vi "Прием ОС (SubVI).vi"(10 "Адрес ОУ":u8, 11 "RX Data":bool[](array[boolean])) -> (2 "Признаки":bool[](array[boolean]), 3 "Ошибка ОС":bool)   [LabVIEW 2015]
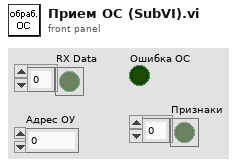
[diagram p1: front panel]
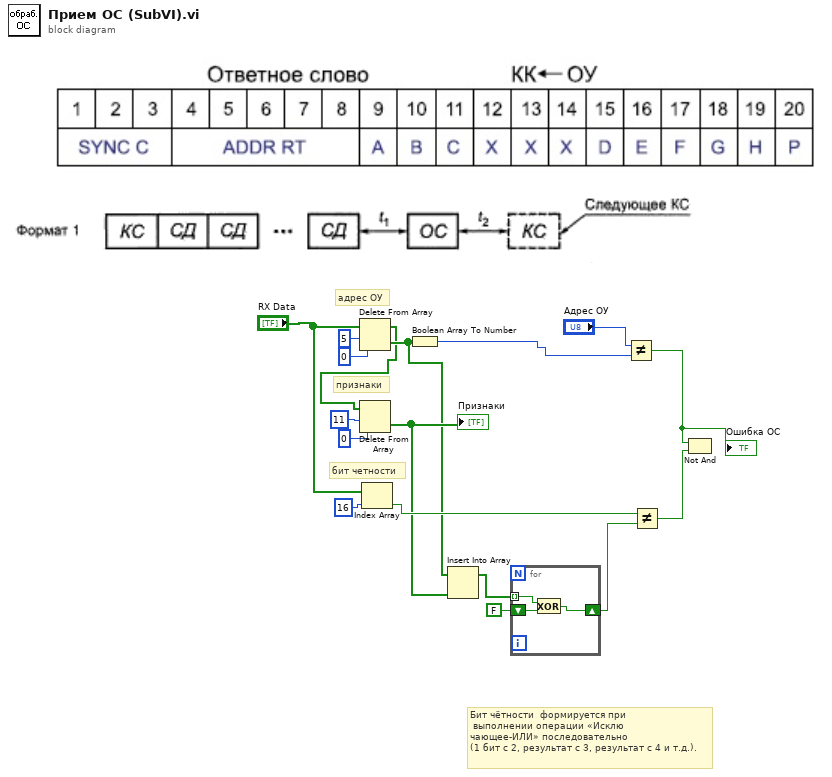
[diagram p0: block diagram]
diagram:
  # "Бит чётности  формируется при\n выполнении операции «Исклю\nчающее-ИЛИ» последовательно \n(1 бит с 2, результат с 3, результат с 4 и т.д.)."
  # "бит четности"
  # "признаки"
  # "адрес ОУ"
  n1 = Delete From Array(array="RX Data", length=5, index=0) -> (deleted portion=w11:bool[], array with subset deleted=w3:bool[])
  n2 = Delete From Array(array=w3, length=11, index=0) -> (deleted portion=w12:bool[])  [unwired: 1 out]
  "Признаки" <- w12
  n3 = Index Array(array="RX Data", index=16 ("length")) -> (element=w14:bool)
  n4 = Boolean Array To Number(Boolean array=w11) -> (number=w16:u32)
  n5 = Insert Into Array(array=w11, new element=w12) -> (w10:bool[])  [unwired: 1 in]
  n6 = for {
    tunnel: w10 -> [w20] mode=indexing
    shift-right: [w19] -> w13
    shift-left: FALSE -> [w18]
    n7 = Exclusive Or(1:w18, 2:w20) -> (0:w19:bool)
  }
  n8 = Not Equal?(x="Адрес ОУ", y=w16) -> (x != y?=w1:bool)
  "Ошибка ОС" <- w1
  n9 = Not Equal?(x=w14, y=w13) -> (x != y?=w17:bool)
  n10 = Not And(1:w17, 2:w1) -> ()  [unwired: 1 out]
